vi "UpAndDownDecimal.vi"() -> ()   [LabVIEW 2015]
panel:
  in  "Down Button":bool
  in  "Stop Button":bool
  out "bottom right":bool
  out "top right":bool
  out "bottom left":bool
  out "Top":bool
  out "Center":bool
  out "top left":bool
  out "Bottom":bool
  # "Count Up"
  # "Count Down"
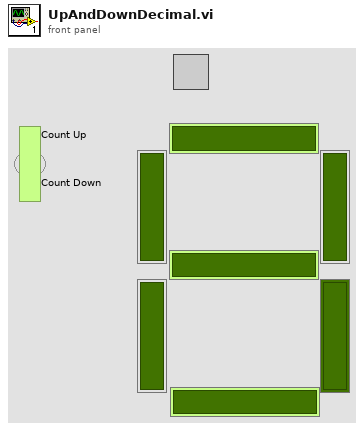
[diagram p1: front panel]
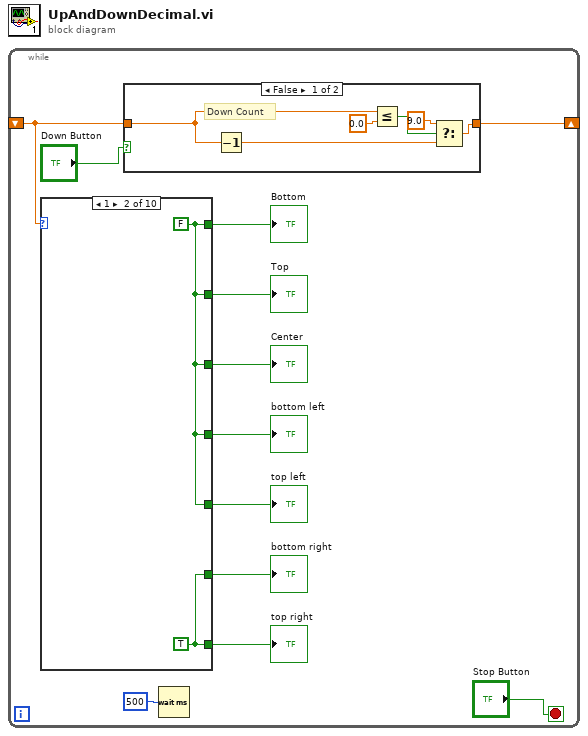
[diagram p0: block diagram]
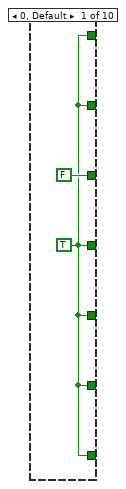
[diagram p2: hidden frame]
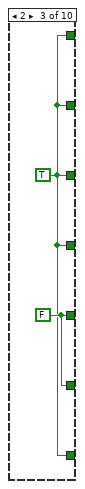
[diagram p3: hidden frame]
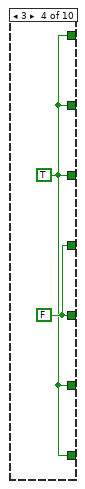
[diagram p4: hidden frame]
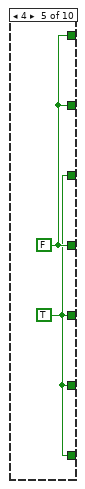
[diagram p5: hidden frame]
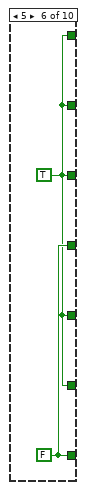
[diagram p6: hidden frame]
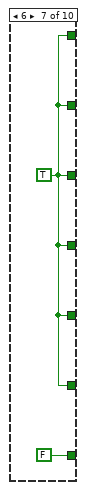
[diagram p7: hidden frame]
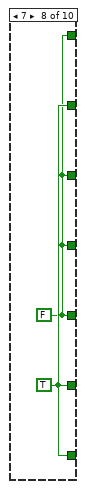
[diagram p8: hidden frame]
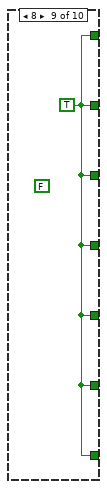
[diagram p9: hidden frame]
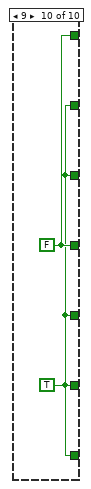
[diagram p10: hidden frame]
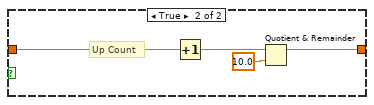
[diagram p11: hidden frame]
diagram:
  n1 = while {
    shift-right: [w2] -> _
    shift-left: _ -> [w1]
    stop <- "Stop Button" stop-if-true
    n2 = case shown="1" w1 {
      tunnel: [w13 w15 w17 w19 w22 w23 w25 w28 w29 w30] -> w9
      tunnel: [w13 w15 w18 w20 w21 w23 w25 w27 w29 w30] -> w8
      tunnel: [w13 w16 w17 w19 w21 w24 FALSE w28 w29 w30] -> w7
      tunnel: [FALSE w15 w17 w19 w21 w23 w25 w27 w29 w30] -> w6
      tunnel: [w13 w15 w17 w20 w22 w24 w25 w27 w29 w31] -> w5
      tunnel: [w13 w16 w18 w19 w21 w23 w25 w28 w29 w30] -> w4
      tunnel: [w13 w15 w17 w19 w22 w23 w25 w27 w29 w31] -> w3
      frame 0, Default {
        w13 = TRUE
      }
      frame 1 {
        w15 = FALSE
        w16 = TRUE
      }
      frame 2 {
        w18 = FALSE
        w17 = TRUE
      }
      frame 3 {
        w20 = FALSE
        w19 = TRUE
      }
      frame 4 {
        w22 = FALSE
        w21 = TRUE
      }
      frame 5 {
        w24 = FALSE
        w23 = TRUE
      }
      frame 6 {
        w25 = TRUE
      }
      frame 7 {
        w27 = FALSE
        w28 = TRUE
      }
      frame 8 {
        (unwired) FALSE
        w29 = TRUE
      }
      frame 9 {
        w31 = FALSE
        w30 = TRUE
      }
    }
    "Bottom" <- w3
    "top left" <- w8
    "Center" <- w6
    "Top" <- w9
    "bottom left" <- w5
    "top right" <- w7
    "bottom right" <- w4
    n3 = case shown="False" "Down Button" {
      tunnel: [w34 w39] -> w2
      tunnel: w1 -> [w32 w38]
      frame False {
        # "Down Count"
        n4 = Decrement(x=w32) -> (x-1=w33:dbl)
        n5 = Less Or Equal?(x=w32, y=0.0) -> (x <= y?=w36:bool)
        n6 = Select(t=9.0, s=w36, f=w33) -> (s? t:f=w34:dbl)
      }
      frame True {
        # "Up Count"
        n7 = Increment(x=w38) -> (x+1=w40:dbl)
        n8 = Quotient & Remainder(x=w40, y=10.0 ("floor(x/y)")) -> (x-y*floor(x/y)=w39:dbl)  [unwired: 1 out]
      }
    }
    n9 = Wait (ms)(milliseconds to wait=u32 500 ("millisecond timer value")) -> ()  [unwired: 1 out]
  }
